vi "GitCheckSaveNeeded.vi"(7 "error in (no error)":errorcluster, 8 "Save Repo Path":path=path "", 9 "Save Cluster":T1 {"Select Layout" items=["Default"]}, 10 "Git exec":string="git") -> (0 "error out":errorcluster, 1 "Save Repo Path Out":path, 2 "Continue":bool, 3 "Git exec out":string="git")   [LabVIEW 2013]
uses:
  DeviceVIs/Device/Device.lvclass
  <vilib>/Utility/miscctls.llb/LVStringsAndValuesArrayTypeDef_I32.ctl
  VariableManagerCodes/VariableManager/VariableManager.lvclass
  TypeDefs/SaveCluster.ctl
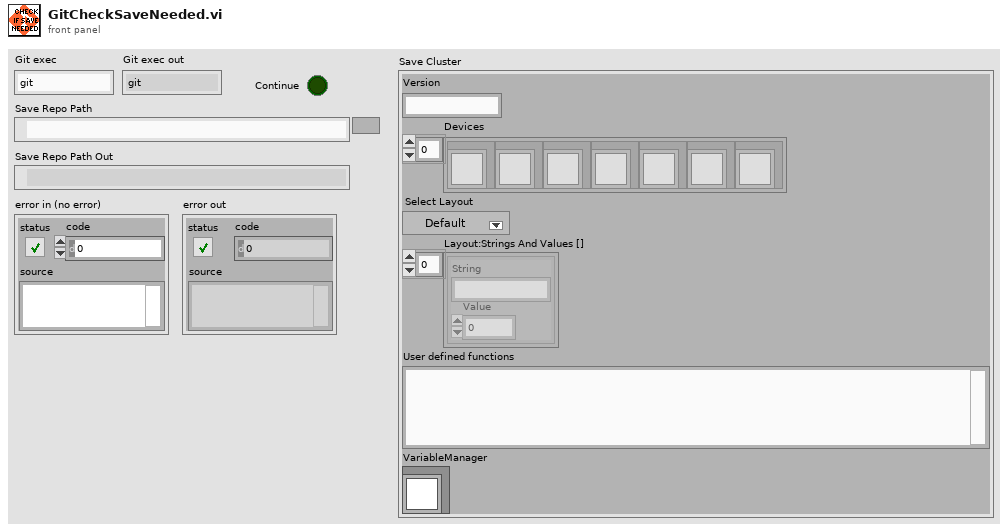
[diagram p1: front panel]
types:
  T1 = typedef "SaveCluster.ctl" = cluster{"Version":string, "Devices":refnum<class "Device.lvclass">[], "Select Layout":i32, "Layout:Strings And Values []":T2, "User defined functions":string, "VariableManager":refnum<class "VariableManager.lvclass">}
  T2 = typedef "LVStringsAndValuesArrayTypeDef_I32.ctl" = cluster{"String":string, "Value":i32}[]
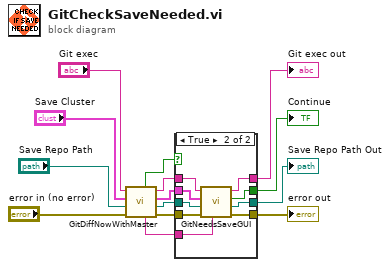
[diagram p0: block diagram]
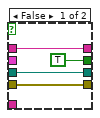
[diagram p2: hidden frame]
diagram:
  n1 = call "GitDiffNowWithMaster.vi"("error in (no error)"="error in (no error)", "Save Repo Path"="Save Repo Path", "Save Cluster"="Save Cluster", "Git exec"="Git exec") -> ("error out"=w4:errorcluster, "Save Repo Path Out"=w6:path, "Save Cluster Out"=w2:T1, "Git exec out"=w7:string, "Diff Output"=w1:string, "Differ"=w10:bool)  [unwired: 2 in]
  n2 = case shown="True" w10 {
    tunnel: [TRUE w20] -> w9
    tunnel: [w17 w27] -> w8
    tunnel: w7 -> [w17 w21]
    tunnel: w6 -> [w16 w23]
    tunnel: [w16 w19] -> w5
    tunnel: w4 -> [w15 w24]
    tunnel: [w15 w26] -> w3
    tunnel: w2 -> [_ w22]
    tunnel: w1 -> [_ w25]
    frame False {
    }
    frame True {
      n3 = call "GitNeedsSaveGUI.vi"("Diff Input"=w25, "error in (no error)"=w24, "Save Repo Path"=w23, "Save Cluster"=w22, "Git exec"=w21) -> ("error out"=w26:errorcluster, "Save Repo Path Out"=w19:path, "Continue"=w20:bool, "Git exec out"=w27:string)  [unwired: 3 in]
    }
  }
  "Git exec out" <- w8
  "error out" <- w3
  "Save Repo Path Out" <- w5
  "Continue" <- w9
